vi "Read Bounds.vi"(8 "error in (no error)":errorcluster, 11 "Shape in":refnum<class "Shape.lvclass">) -> (0 "error out":errorcluster, 2 "Bounds":T1, 3 "Shape out":refnum<class "Shape.lvclass">)   [LabVIEW 2017, in "LV Image Editor Framework.lvlib" / "Shape.lvclass"]
uses:
  <vilib>/LIEF/Forms/Shape/Shape.lvclass
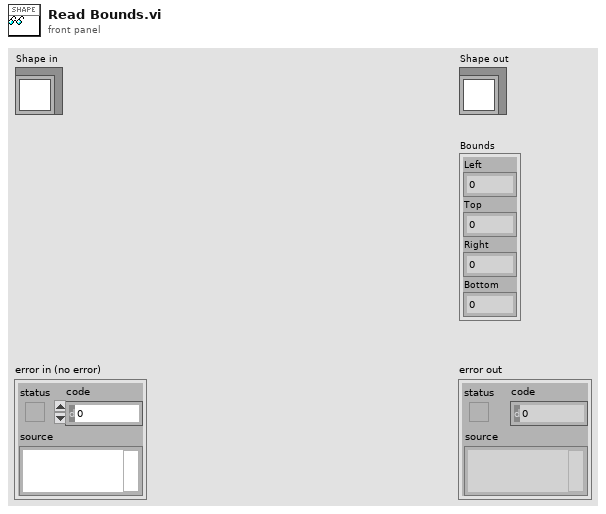
[diagram p1: front panel]
types:
  T1 = cluster{"Left":i32, "Top":i32, "Right":i32, "Bottom":i32}
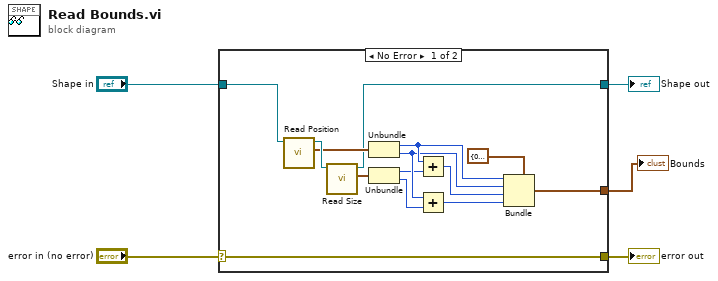
[diagram p0: block diagram]
diagram:
  n1 = case shown="No Error" "error in (no error)" {
    selector: "error in (no error)" -> [w19 w20]
    tunnel: [w19 w20] -> w4
    tunnel: [w7 w21] -> w2
    tunnel: "Shape in" -> [w8 w21]
    tunnel: [w6 _] -> w1
    frame No Error {
      n2 = call-dynamic "Read Position.vi"("Shape in"=w8) -> ("Position"=w14:cluster{"Left":i32, "Top":i32}, "Shape out"=w15:refnum<class "Shape.lvclass">)  [unwired: 8 in, 1 out]
      n3 = call-dynamic "Read Size.vi"("Shape in"=w15) -> ("Size"=w13:cluster{"Width":i32, "Height":i32}, "Shape out"=w7:refnum<class "Shape.lvclass">)  [unwired: 8 in, 1 out]
      n4 = Unbundle(w14) -> ("Left"=w12:i32, "Top"=w11:i32)
      n5 = Unbundle(w13) -> ("Width"=w10:i32, "Height"=w9:i32)
      n6 = Add(x=w12, y=w10) -> (x+y=w18:i32)
      n7 = Add(x=w11, y=w9) -> (x+y=w17:i32)
      n8 = Bundle(cluster=T1 {"Left"=0, "Top"=0, "Right"=0, "Bottom"=0} ("output cluster"), "Left"=w12, "Top"=w11, "Right"=w18, "Bottom"=w17) -> (w6:T1)
    }
    frame Error {
    }
  }
  "error out" <- w4
  "Shape out" <- w2
  "Bounds" <- w1
